vi "Queue Sender.vi"() -> ()   [LabVIEW 2009]
uses:
  Element.ctl
  <vilib>/Platform/TimedLoop/XDataNode/XDataNode.xnode
  <vilib>/Platform/TimedLoop/XDataNode/loadlvalarms.vi
  <vilib>/Platform/TimedLoop/XDataNode/timing_clust.ctl
  <vilib>/Platform/TimedLoop/XDataNode/nitl_modes.ctl
  <vilib>/Platform/TimedLoop/XDataNode/wakeup.ctl
  <vilib>/Platform/TimedLoop/XDataNode/XDNodeRunTimeDep.lvlib
panel:
  in  "String 2":string
  in  "String 1":string="123123"
  in  "OK Button":bool
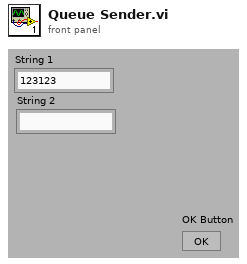
[diagram p1: front panel]
types:
  T1 = typedef "Element.ctl" = cluster{"String 1":string, "String 2":string, "Numeric":dbl}
  T2 = typedef "XDNodeRunTimeDep.lvlib/timing_clust.ctl" = cluster{"Expected End [f-1]":u64, "Actual End [f-1]":u64, "Finished Late? [f-1]":bool, "Expected End [i-1]":u64, "Actual End [i-1]":u64, "Finished Late? [i-1]":bool, "Expected Start [i]":u64, "Actual Start [i]":u64, "Expected Start [f]":u64, "Actual Start [f]":u64, "Source Name":string, "Structure Name":string, "Period":i64, "Deadline":i64, "Offset":i64, "Start":i64, "Priority":i32, "Timeout":i32, "Mode":T3, "Wakeup Reason":T4, "Error":errorcluster, "Source Type":string, "Secondary Source Type":string, "Global End Time":u64, "Global Start Time":u64, "Frame Duration":u64, "Iteration Duration":u64, "Assigned CPU":i32, "I/O Scan Engine Mode":u32}
  T3 = typedef "XDNodeRunTimeDep.lvlib/nitl_modes.ctl" = enum32{"No Change", "Process missed periods, maintain original phase", "Discard missed periods, maintain original phase", "Process missed periods, ignore original phase", "Discard missed periods, ignore original phase"}
  T4 = typedef "XDNodeRunTimeDep.lvlib/wakeup.ctl" = enum32{"Normal", "Aborted", "Asynchronous wakeup", "Timing source error", "Timed loop error", "Timeout"}
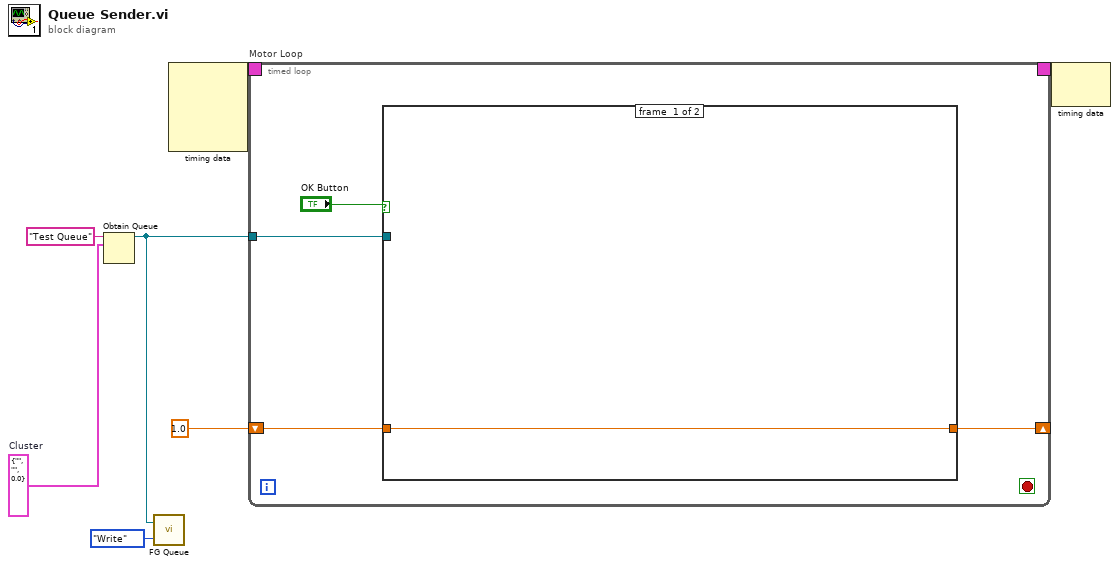
[diagram p0: block diagram]
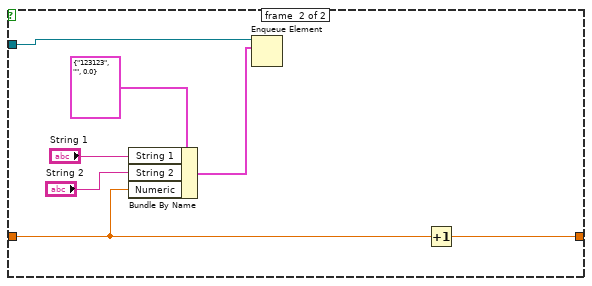
[diagram p2: hidden frame]
diagram:
  w4 = T1 {"String 1"="", "String 2"="", "Numeric"=0.0}  # Cluster
  n1 = Obtain Queue(name (unnamed)="Test Queue", element data type=w4) -> (queue out=w1:refnum<queue>)  [unwired: 3 in, 2 out]
  n2 = call "FG Queue.vi"("FG Action"=enum16{"Read", "Write"}."Write", "queue in"=w1) -> ()  [unwired: 1 in, 1 out]
  n3 = node-c288() -> (w7:T2)  [unwired: 4 in]
  n4 = timed-loop "Motor Loop" {
    timing: w7 -> [_]
    timing-out: [_] -> w6
    tunnel: w1 -> [w10]
    shift-right: [w8] -> _
    shift-left: 1.0 ("Numeric") -> [w9]
    stop <- _ stop-if-true
    n5 = case shown="True" "OK Button" {
      tunnel: w10 -> [_ w19]
      tunnel: w9 -> [w12 w15]
      tunnel: [w12 w14] -> w8
      frame #0 {
      }
      frame #1 {
        n6 = Bundle By Name(cluster=T1 {"String 1"="123123", "String 2"="", "Numeric"=0.0} ("Cluster"), "String 1"="String 1", "String 2"="String 2", "Numeric"=w15) -> (w13:T1)
        n7 = Enqueue Element(queue=w19, element=w13) -> ()  [unwired: 2 in, 3 out]
        n8 = Increment(x=w15) -> (x+1=w14:dbl)
      }
    }
  }
  n9 = node-c288(w6) -> ()  [unwired: 1 out]
